vi "removeItem.vi"(8 "error in (no error)":errorcluster, 10 "Key":string, 11 "HashMap in":refnum<class "HashMap.lvclass">) -> (0 "error out":errorcluster, 3 "HashMap out":refnum<class "HashMap.lvclass">)   [LabVIEW 2017, in "HashMap.lvclass"]
uses:
  <userlib>/836-Library/Data_Structures/HashMap/HashMap.lvclass
  <userlib>/836-Library/Data_Structures/HashMap/HashMap.lvclass/HashMap.ctl
  <vilib>/Utility/error.llb/Error Cluster From Error Code.vi
  <vilib>/ErrorRing/Error Ring.xnode
  <userlib>/836-Library/Data_Structures/Bucket/Bucket.lvclass
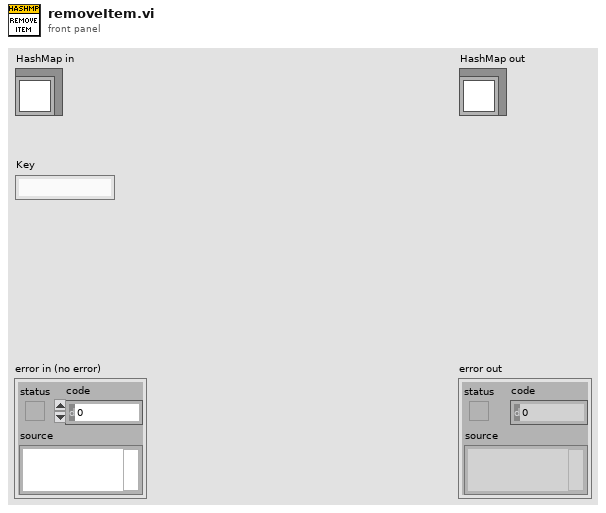
[diagram p1: front panel]
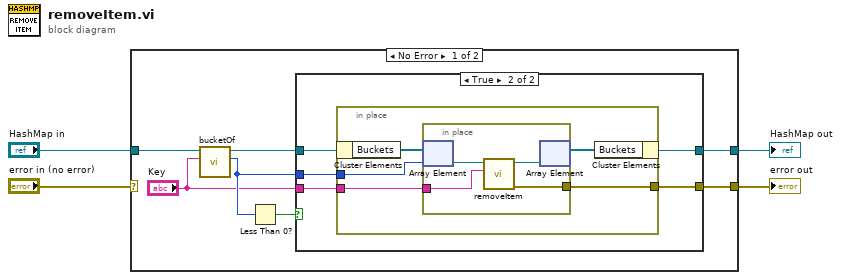
[diagram p0: block diagram]
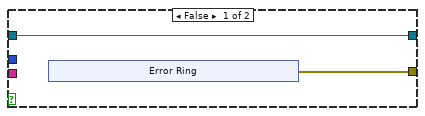
[diagram p2: hidden frame]
diagram:
  n1 = case shown="No Error" "error in (no error)" {
    selector: "error in (no error)" -> [_ w34]
    tunnel: [w5 w34] -> w3
    tunnel: [w6 w33] -> w1
    tunnel: "HashMap in" -> [w11 w33]
    frame No Error {
      n2 = call <userlib>:"bucketOf.vi"("Key"="Key", "HashMap in"=w11) -> ("Bucket Index"=w8:i32, "HashMap out"=w9:refnum<class "HashMap.lvclass">)  [unwired: 7 in, 1 out]
      n3 = Less Than 0?(x=w8) -> (x < 0?=w10:bool)
      n4 = case shown="True" w10 {
        tunnel: w9 -> [w13 w23]
        tunnel: w8 -> [_ w22]
        tunnel: [w12 w21] -> w5
        tunnel: "Key" -> [_ w20]
        tunnel: [w13 w19] -> w6
        frame False {
          n5 = xnode "Error Ring"() -> ("error out"=w12:errorcluster)
        }
        frame True {
          n6 = in-place {
            in-place-border: w22 -> [w27]
            in-place-border: [w26] -> w21
            in-place-border: w20 -> [w25]
            n7 = in-place-cluster #1(w23) -> ("Buckets"=w28:refnum<class "Bucket.lvclass">[])
            n8 = in-place {
              in-place-border: [w30] -> w26
              in-place-border: w25 -> [w29]
              n9 = in-place-array #2(w28, w27) -> (w32:refnum<class "Bucket.lvclass">)
              n10 = call <userlib>:"removeItem.vi"("Key"=w29, "Bucket in"=w32) -> ("error out"=w30:errorcluster, "Bucket out"=w31:refnum<class "Bucket.lvclass">)  [unwired: 8 in]
              n11 = in-place-array #2(w31) -> (w24:refnum<class "Bucket.lvclass">[])  [unwired: 1 out]
            }
            n12 = in-place-cluster #1("Buckets"=w24) -> (w19:refnum<class "HashMap.lvclass">)
          }
        }
      }
    }
    frame Error {
    }
  }
  "error out" <- w3
  "HashMap out" <- w1
